vi "Read ExecutionState.vi"(8 "error in (no error)":errorcluster, 11 "ExecutionControls in":refnum<class "ExecutionControls.lvclass">) -> (0 "error out":errorcluster, 1 "Paused = T":bool, 2 "Running = T":bool, 3 "ExecutionControls out":refnum<class "ExecutionControls.lvclass">)   [LabVIEW 2018, in "ExecutionControls.lvclass"]
uses:
  ExecutionControls.lvclass
  ExecutionControls.lvclass/ExecutionControls.ctl
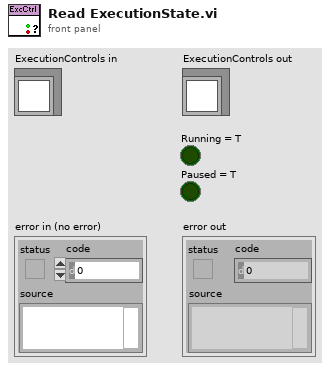
[diagram p1: front panel]
types:
  T1 = enum8{"Enabled", "Disabled", "Disabled and Grayed Out"}
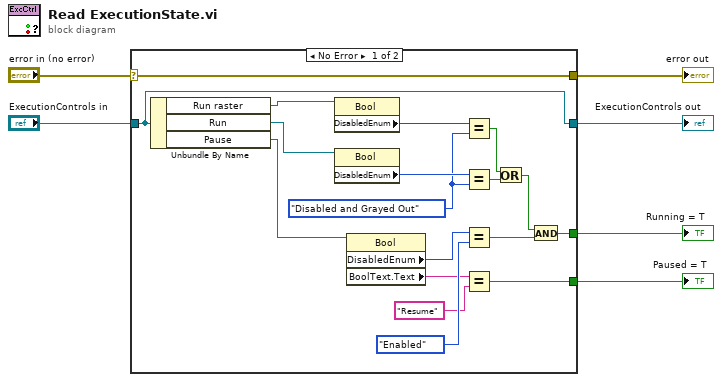
[diagram p0: block diagram]
diagram:
  n1 = case shown="No Error" "error in (no error)" {
    selector: "error in (no error)" -> [w24 w26]
    tunnel: [w24 w26] -> w5
    tunnel: [w23 w25] -> w3
    tunnel: "ExecutionControls in" -> [w23 w25]
    tunnel: [w14 _] -> w2
    tunnel: [w13 _] -> w1
    frame No Error {
      w10 = T1."Disabled and Grayed Out" ("Disabled")
      n2 = Unbundle By Name(w23) -> ("Run raster"=w12:refnum<vi>, "Run"=w22:refnum<vi>, "Pause"=w18:refnum<vi>)
      n3 = property class="Bool"(reference=w12) -> ("DisabledEnum"=w11:T1)  [unwired: 1 in, 2 out]
      n4 = property class="Bool"(reference=w22) -> ("DisabledEnum"=w21:T1)  [unwired: 1 in, 2 out]
      n5 = property class="Bool"(reference=w18) -> ("DisabledEnum"=w19:T1, "BoolText.Text"=w17:string)  [unwired: 1 in, 2 out]
      n6 = Equal?(x=w11, y=w10) -> (x = y?=w8:bool)
      n7 = Equal?(x=w21, y=w10) -> (x = y?=w9:bool)
      n8 = Equal?(x=w19, y=T1."Enabled" ("Disabled")) -> (x = y?=w15:bool)
      n9 = Equal?(x=w17, y="Resume" ("Boolean Text.Text")) -> (x = y?=w13:bool)
      n10 = Or(x=w8, y=w9) -> (x .or. y?=w7:bool)
      n11 = And(x=w7, y=w15) -> (x .and. y?=w14:bool)
    }
    frame Error {
    }
  }
  "error out" <- w5
  "ExecutionControls out" <- w3
  "Running = T" <- w2
  "Paused = T" <- w1
